vi "insertOvenLot.vi"(8 "error in (no error)":errorcluster, 10 "lot list":string, 11 "connection reference":T1) -> (0 "error out":errorcluster, 3 "connection reference out":T1)   [LabVIEW 2012]
uses:
  <vilib>/addons/database/Connection.llb/Conn ObjectReference.ctl
  <vilib>/addons/database/Connection.llb/Conn Execute.vi
  <vilib>/addons/database/Recordset.llb/Rec Fetch Integer Data (R).vi
  <vilib>/addons/database/Recordset.llb/Rec Destroy - Connection.vi
  <vilib>/addons/database/NI_Database_API.lvlib
panel:
  in  "input cluster":cluster{"rc":string, "lots":string}
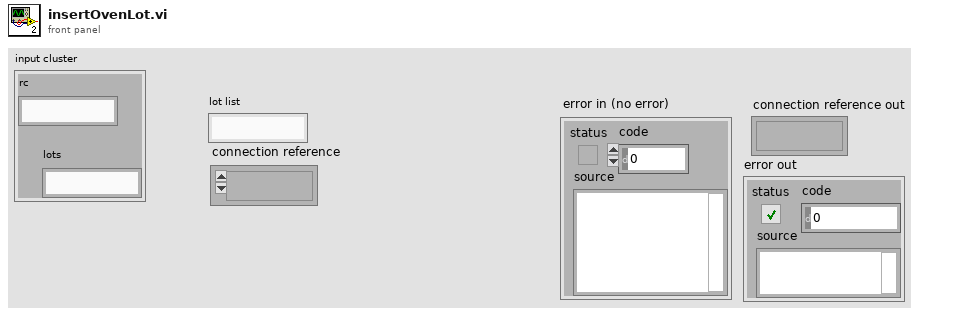
[diagram p1: front panel]
types:
  T1 = typedef "NI_Database_API.lvlib/Conn ObjectReference.ctl" = refnum<k1>
  T2 = typedef "NI_Database_API.lvlib/Rec ObjectReference.ctl" = refnum<k1>
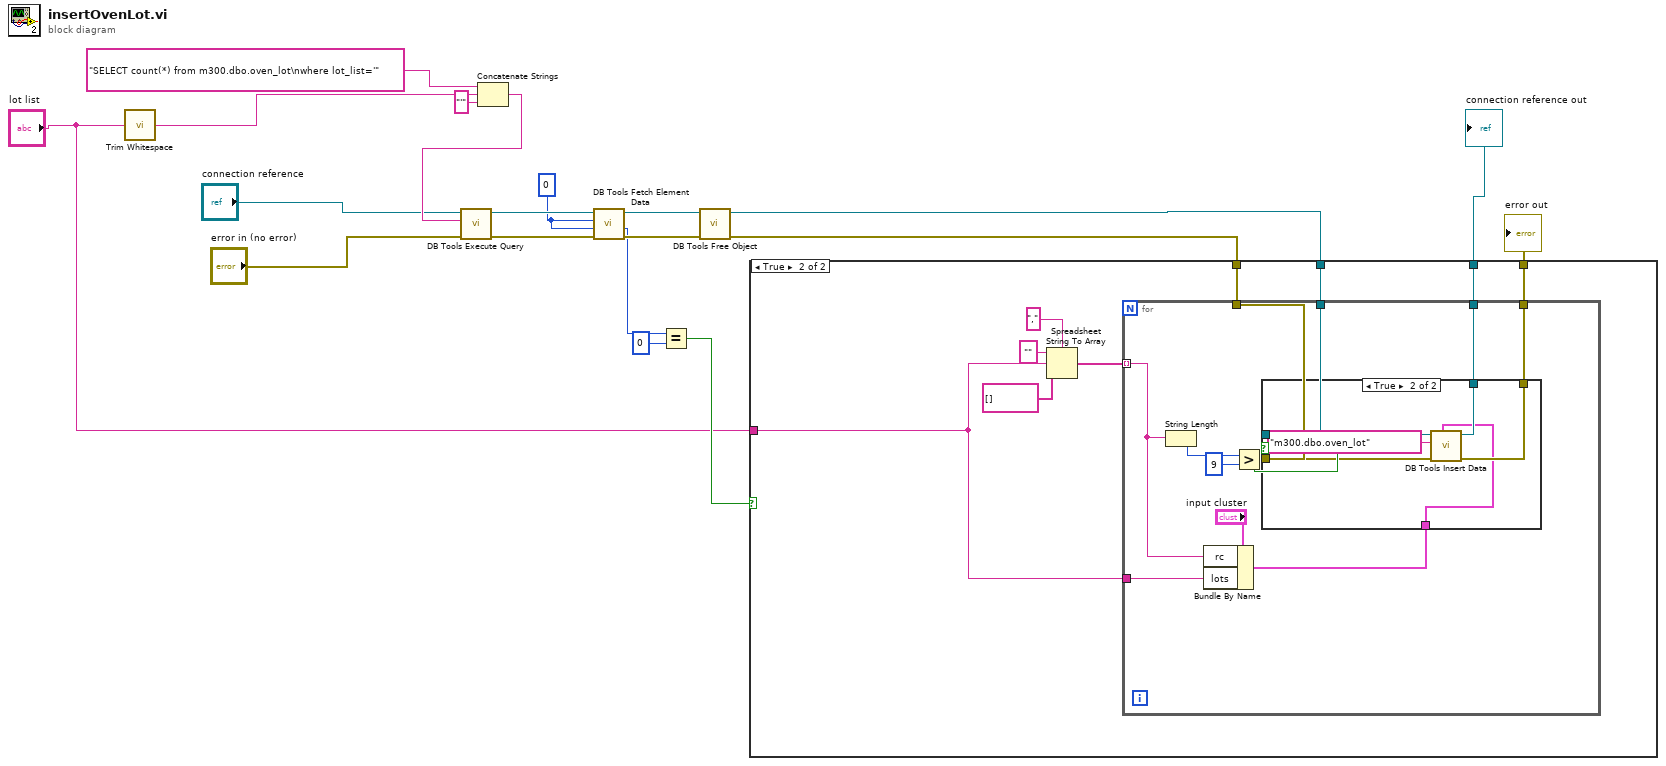
[diagram p0: block diagram]
diagram:
  w9 = 0
  n1 = call <vilib>:"Trim Whitespace.vi"("string"="lot list") -> ("trimmed string"=w11:string)  [unwired: 1 in]
  n2 = Concatenate Strings("SELECT count(*) from m300.dbo.oven_lot\nwhere lot_list='" ("SQL query"), w11, "'" ("string")) -> (w10:string)
  n3 = call-poly <vilib>:"DB Tools Execute Query.vi"("error in (no error)"="error in (no error)", "SQL query"=w10, "connection reference"="connection reference") -> ("error out"=w18:errorcluster, "recordset reference"=w19:T2)  [unwired: 5 in]
  n4 = call-poly <vilib>:"DB Tools Fetch Element Data.vi"("error in (no error)"=w18, "type"=w9, "column index"=w9, "recordset reference"=w19) -> ("error out"=w16:errorcluster, "data"=w8:i32, "recordset reference out"=w17:T2)  [unwired: 3 in]
  n5 = Equal?(x=w8, y=0) -> (x = y?=w6:bool)
  n6 = call-poly <vilib>:"DB Tools Free Object.vi"("error in (no error)"=w16, "recordset reference"=w17) -> ("error out"=w14:errorcluster, "connection reference"=w15:T1)  [unwired: 8 in]
  n7 = case shown="True" w6 {
    tunnel: w15 -> [w21 w30]
    tunnel: w14 -> [w20 w29]
    tunnel: [w21 w28] -> w2
    tunnel: [w20 w27] -> w1
    tunnel: "lot list" -> [_ w22]
    frame False {
    }
    frame True {
      n8 = Spreadsheet String To Array(delimiter (Tab)=",", format string="", spreadsheet string=w22, array type (2D Dbl)=string[] []) -> (array=w23:string[])
      n9 = for {
        tunnel: w23 -> [w33] mode=indexing
        tunnel: w30 -> [w39]
        tunnel: w29 -> [w38]
        tunnel: [w37] -> w28
        tunnel: [w36] -> w27
        tunnel: w22 -> [w32]
        n10 = String Length(string=w33) -> (length=w41:i32)
        n11 = Bundle By Name(cluster="input cluster", "rc"=w33, "lots"=w32) -> (w31:cluster{"rc":string, "lots":string})
        n12 = Greater?(x=w41, y=9) -> (0:w35:bool)
        n13 = case shown="True" w35 {
          tunnel: w39 -> [w43 w49]
          tunnel: w38 -> [w42 w48]
          tunnel: [w43 w47] -> w37
          tunnel: [w42 w46] -> w36
          tunnel: w31 -> [_ w44]
          frame False {
          }
          frame True {
            n14 = call <vilib>:"DB Tools Insert Data.vi"("data"=w44, "error in (no error)"=w48, "table"="m300.dbo.oven_lot", "connection reference"=w49) -> ("error out"=w46:errorcluster, "connection reference out"=w47:T1)  [unwired: 6 in]
          }
        }
      }
    }
  }
  "connection reference out" <- w2
  "error out" <- w1
